vi "cDAQ UI - Handle Images.vi"(8 "error in":errorcluster, 11 "Current VI Path Out":path) -> (0 "error out":errorcluster, 2 "Images Out":picture[](array[picture]), 3 "Dup Path Out":path, 5 "Nr of Images Out":i32)   [LabVIEW 2011]
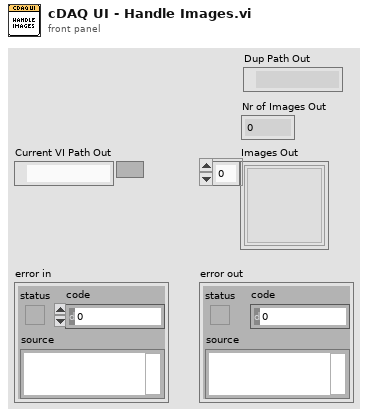
[diagram p1: front panel]
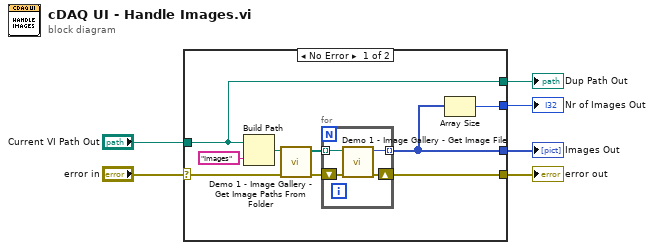
[diagram p0: block diagram]
diagram:
  n1 = case shown="No Error" "error in" {
    selector: "error in" -> [w8 w20]
    tunnel: [w15 w20] -> w6
    tunnel: "Current VI Path Out" -> [w7 _]
    tunnel: [w10 _] -> w4
    tunnel: [w9 _] -> w3
    tunnel: [w7 _] -> w1
    frame No Error {
      n2 = Build Path(base path=w7, name or relative path="Images") -> (appended path=w14:path)
      n3 = call "Demo 1 - Image Gallery - Get Image Paths From Folder.vi"("Error In"=w8, "Image Folder Path In"=w14) -> ("Error Out"=w11:errorcluster, "Image Paths Out"=w12:path[])  [unwired: 8 in]
      n4 = for {
        tunnel: w12 -> [w18] mode=indexing
        shift-right: [w17] -> w15
        shift-left: w11 -> [w19]
        tunnel: [w16] -> w10 mode=indexing
        n5 = call "Demo 1 - Image Gallery - Get Image File.vi"("Error In"=w19, "Image Path In"=w18) -> ("Error Out"=w17:errorcluster, "Image Out"=w16:picture)  [unwired: 8 in]
      }
      n6 = Array Size(array=w10) -> (size(s)=w9:i32)
    }
    frame Error {
    }
  }
  "error out" <- w6
  "Images Out" <- w4
  "Nr of Images Out" <- w3
  "Dup Path Out" <- w1
